vi "main.vi"() -> ()   [LabVIEW 2018, in "InterpreterPatternDemo.lvclass"]
uses:
  InterpreterPatternDemo.lvclass
  ConsoleOut/Print Options.ctl
  OrExpression Class/OrExpression.lvclass
  AndExpression Class/AndExpression.lvclass
panel:
  out "error out":errorcluster
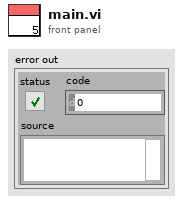
[diagram p1: front panel]
types:
  T1 = typedef "Print Options.ctl" = enum16{"Create", "Get Reference", "Print", "Print Header", "Close"}
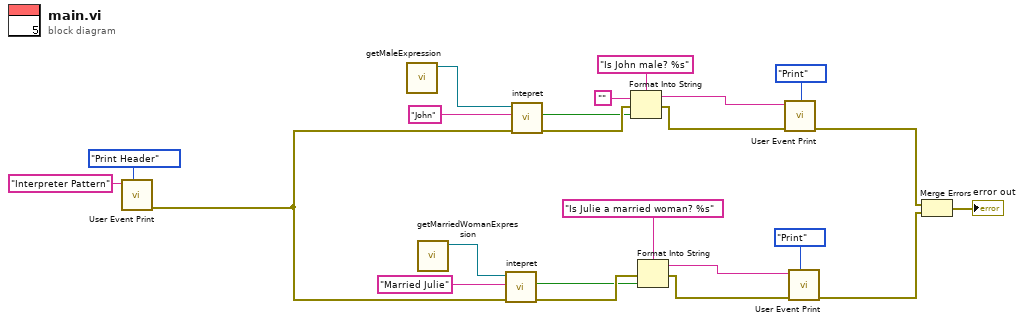
[diagram p0: block diagram]
diagram:
  n1 = call "User Event Print.vi"("Options"=Print_Options."Print Header", "String to Print"="Interpreter Pattern") -> ("error out"=w8:errorcluster)  [unwired: 8 in, 1 out]
  n2 = call "getMaleExpression.vi"() -> ("OrExpression"=w23:refnum<class "OrExpression.lvclass">)  [unwired: 11 in]
  n3 = call "getMarriedWomanExpression.vi"() -> ("AndExpression"=w18:refnum<class "AndExpression.lvclass">)  [unwired: 11 in]
  n4 = call-dynamic "intepret.vi"("error in (no error)"=w8, "context"="Married Julie", "AndExpression in"=w18) -> ("error out"=w5:errorcluster, "result"=w4:bool)  [unwired: 6 in, 1 out]
  n5 = call-dynamic "intepret.vi"("error in (no error)"=w8, "context"="John", "OrExpression in"=w23) -> ("error out"=w7:errorcluster, "result"=w6:bool)  [unwired: 6 in, 1 out]
  n6 = Format Into String(format string="Is John male? %s", initial string="", error in=w7, w6) -> (resulting string=w11:string, error out=w12:errorcluster)
  n7 = Format Into String(format string="Is Julie a married woman? %s", error in=w5, w4) -> (resulting string=w14:string, error out=w13:errorcluster)  [unwired: 1 in]
  n8 = call "User Event Print.vi"("Options"=Print_Options."Print", "error in (no error)"=w12, "String to Print"=w11) -> ("error out"=w3:errorcluster)  [unwired: 7 in, 1 out]
  n9 = call "User Event Print.vi"("Options"=Print_Options."Print", "error in (no error)"=w13, "String to Print"=w14) -> ("error out"=w2:errorcluster)  [unwired: 7 in, 1 out]
  n10 = Merge Errors(w3, w2) -> (→"error out":errorcluster)
